vi "intake.vi"(9 "Current Time":i32, 10 "Ball in elevator":bool, 11 "Top Limit switch":bool) -> (3 "Operation finished":bool)   [LabVIEW 2015]
uses:
  Robot Global Data.vi
panel:
  in  "Ball At Bottom of elevator":bool
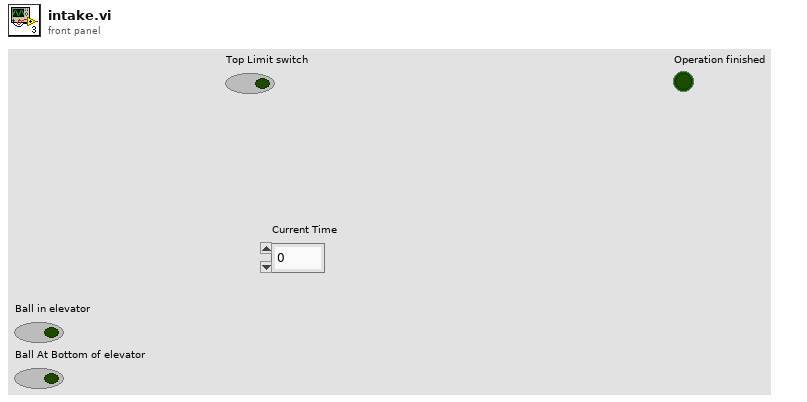
[diagram p1: front panel]
types:
  T1 = enum16{"nothing", "intaketotop", "eject ball", "load ball to shooter", "intaketobottom"}
  T2 = typedef "WPI_MotorControlDeviceRef.ctl" = cluster{"DeviceStatus":errorcluster, "Type":T3, "PWM":cluster{"PWM Channel":T4, "DeadBand":T5}, "CAN":cluster{"Device Number":u8, "Control Mode":T6, "Semaphore":T7, "Max Vout":dbl, "TalonSRX Control Mode":T8}, "Invert":bool}
  T3 = typedef "WPI_MotorControlType.ctl" = enum16{"PWM", "CAN", "CANTalonSRX"}
  T4 = typedef "FPGA_DIOPWMChannel.ctl" = enum8{"PWM 0", "PWM 1", "PWM 2", "PWM 3", "PWM 4", "PWM 5", "PWM 6", "PWM 7", "PWM 8", "PWM 9", "PWM MXP 0", "PWM MXP 1", "PWM MXP 2", "PWM MXP 3", "PWM MXP 4", "PWM MXP 5", "PWM MXP 6", "PWM MXP 7", "PWM MXP 8", "PWM MXP 9", "Invalid"}
  T5 = typedef "WPI_PWMDeadband.ctl" = cluster{"Name":string, "maxPositivePwm":i32, "minPositivePwm":i32, "centerPwm":i32, "maxNegativePwm":i32, "minNegativePwm":i32, "angularRange":u16}
  T6 = typedef "WPI_CANJaguar_ControlMode.ctl" = enum8{"Percent VBus", "Current", "Speed", "Position", "Voltage"}
  T7 = typedef "Semaphore RefNum" = refnum<k1>
  T8 = typedef "WPI_CANTalonSRX_APIControlMode.ctl" = enum8{"Percent VBus", "Speed", "Position", "Slave", "Unchanged / Invalid", "Voltage Compensation", "Current", "Motion Profile"}
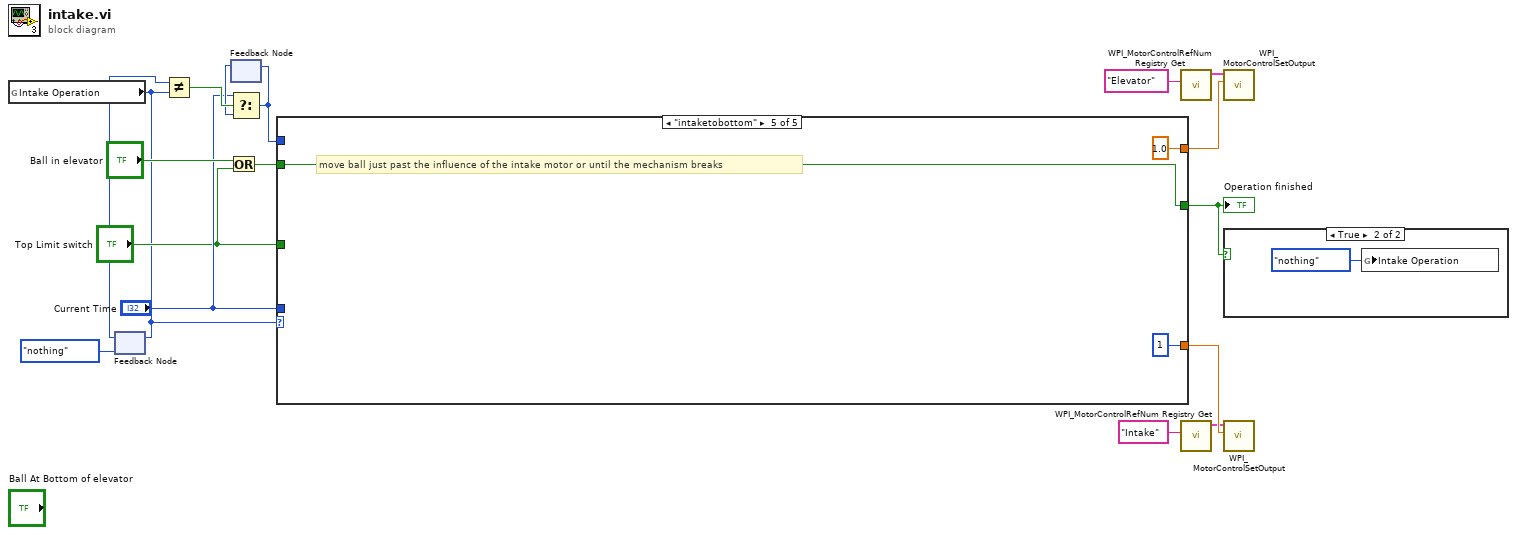
[diagram p0: block diagram]
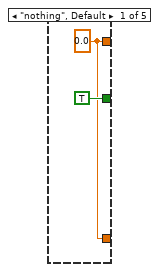
[diagram p3: hidden frame]
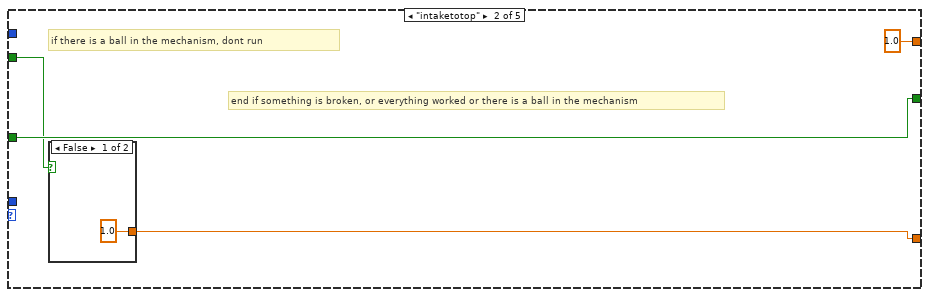
[diagram p4: hidden frame]
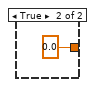
[diagram p5: hidden frame]
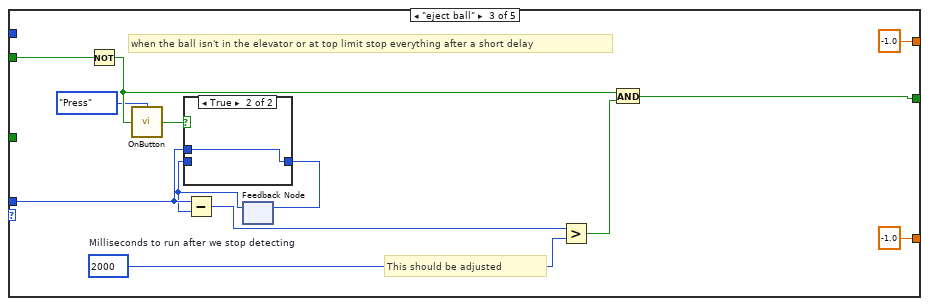
[diagram p6: hidden frame]
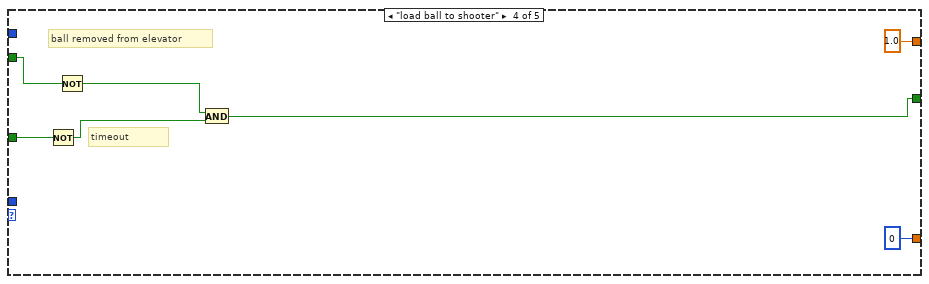
[diagram p8: hidden frame]
diagram:
  n1 = global read "Robot Global Data.vi" "Intake Operation"() -> (w1:T1)
  n2 = feedback #1(T1."nothing" ("Intake Operation")) -> (w14:T1)
  n3 = feedback-in #1(w1) -> ()
  n4 = Not Equal?(x=w14, y=w1) -> (x != y?=w16:bool)
  n5 = Or(x="Ball in elevator", y="Top Limit switch") -> (x .or. y?=w3:bool)
  n6 = feedback #2() -> (w15:i32)  [unwired: 1 in]
  n7 = Select(t="Current Time", s=w16, f=w15) -> (s? t:f=w12:i32)
  n8 = feedback-in #2(w12) -> ()
  n9 = case shown="\"intaketobottom\"" w1 {
    tunnel: "Current Time" -> [_ _ w33 _ _]
    tunnel: [w18 w22 -1.0 ("f") 0 1] -> w9
    tunnel: [TRUE w21 w29 w41 w48] -> w5
    tunnel: [w18 1.0 ("Output") -1.0 ("Output") 1.0 1.0 ("Output")] -> w8
    tunnel: w3 -> [_ w20 w36 w44 w48]
    tunnel: "Top Limit switch" -> [_ w21 _ w45 _]
    tunnel: w12 -> [_ _ _ _ _]
    frame "nothing", Default {
      w18 = 0.0
    }
    frame "intaketotop" {
      # "end if something is broken, or everything worked or there is a ball in the mechanism"
      # "if there is a ball in the mechanism, dont run"
      n10 = case shown="False" w20 {
        tunnel: [1.0 0.0] -> w22
        frame False {
        }
        frame True {
        }
      }
    }
    frame "eject ball" {
      w31 = u32 2000  # Milliseconds to run after we stop detecting
      # "This should be adjusted"
      # "when the ball isn't in the elevator or at top limit stop everything after a short delay"
      n11 = Not(x=w36) -> (.not. x?=w28:bool)
      n12 = call "OnButton.vi"("Button"=w28, "Mode"=enum16{"Press", "Release", "Both"}."Press") -> ("Value"=w27:bool)
      n13 = feedback #3() -> (w32:i32)  [unwired: 1 in]
      n14 = case shown="True" w27 {
        tunnel: [w39 w40] -> w35
        tunnel: w33 -> [_ w40]
        tunnel: w32 -> [w39 _]
        frame False {
        }
        frame True {
        }
      }
      n15 = Subtract(x=w33, y=w32) -> (x-y=w34:i32)
      n16 = feedback-in #3(w35) -> ()
      n17 = Greater?(x=w34, y=w31) -> (0:w30:bool)
      n18 = And(x=w28, y=w30) -> (x .and. y?=w29:bool)
    }
    frame "load ball to shooter" {
      # "ball removed from elevator"
      # "timeout"
      n19 = Not(x=w45) -> (.not. x?=w43:bool)
      n20 = Not(x=w44) -> (.not. x?=w42:bool)
      n21 = And(x=w42, y=w43) -> (x .and. y?=w41:bool)
    }
    frame "intaketobottom" {
      # "move ball just past the influence of the intake motor or until the mechanism breaks"
    }
  }
  "Operation finished" <- w5
  n22 = call <vilib>:"WPI_MotorControlRefNum Registry Get.vi"("refnum name"="Elevator") -> ("MotorControlDevRef"=w7:T2)  [unwired: 9 in, 1 out]
  n23 = call <vilib>:"WPI_MotorControlRefNum Registry Get.vi"("refnum name"="Intake") -> ("MotorControlDevRef"=w6:T2)  [unwired: 9 in, 1 out]
  n24 = call <vilib>:"WPI_MotorControlSetOutput.vi"("Output"=w8, "MotorControlDevRef"=w7) -> ()  [unwired: 7 in, 3 out]
  n25 = case shown="True" w5 {
    frame False {
    }
    frame True {
      n26 = global write "Robot Global Data.vi" "Intake Operation"(T1."nothing" ("Intake Operation")) -> ()
    }
  }
  n27 = call <vilib>:"WPI_MotorControlSetOutput.vi"("Output"=w9, "MotorControlDevRef"=w6) -> ()  [unwired: 7 in, 3 out]
